vi "CommaScriptPaint.vi"(7 "Zoom Factor":sgl, 9 "Starting Pos":i16(slide)=128 scale=340.0..50.0, 10 "string 2":string, 11 "string":string) -> (2 "new picture":picture, 3 "Array":string[](array[string]))   [LabVIEW 2018]
panel:
  out "new picture out":picture
  out "Scaling Factor":dbl=1.07143 format="%#_13g"
  out "Height":u32
  out "Width":u32
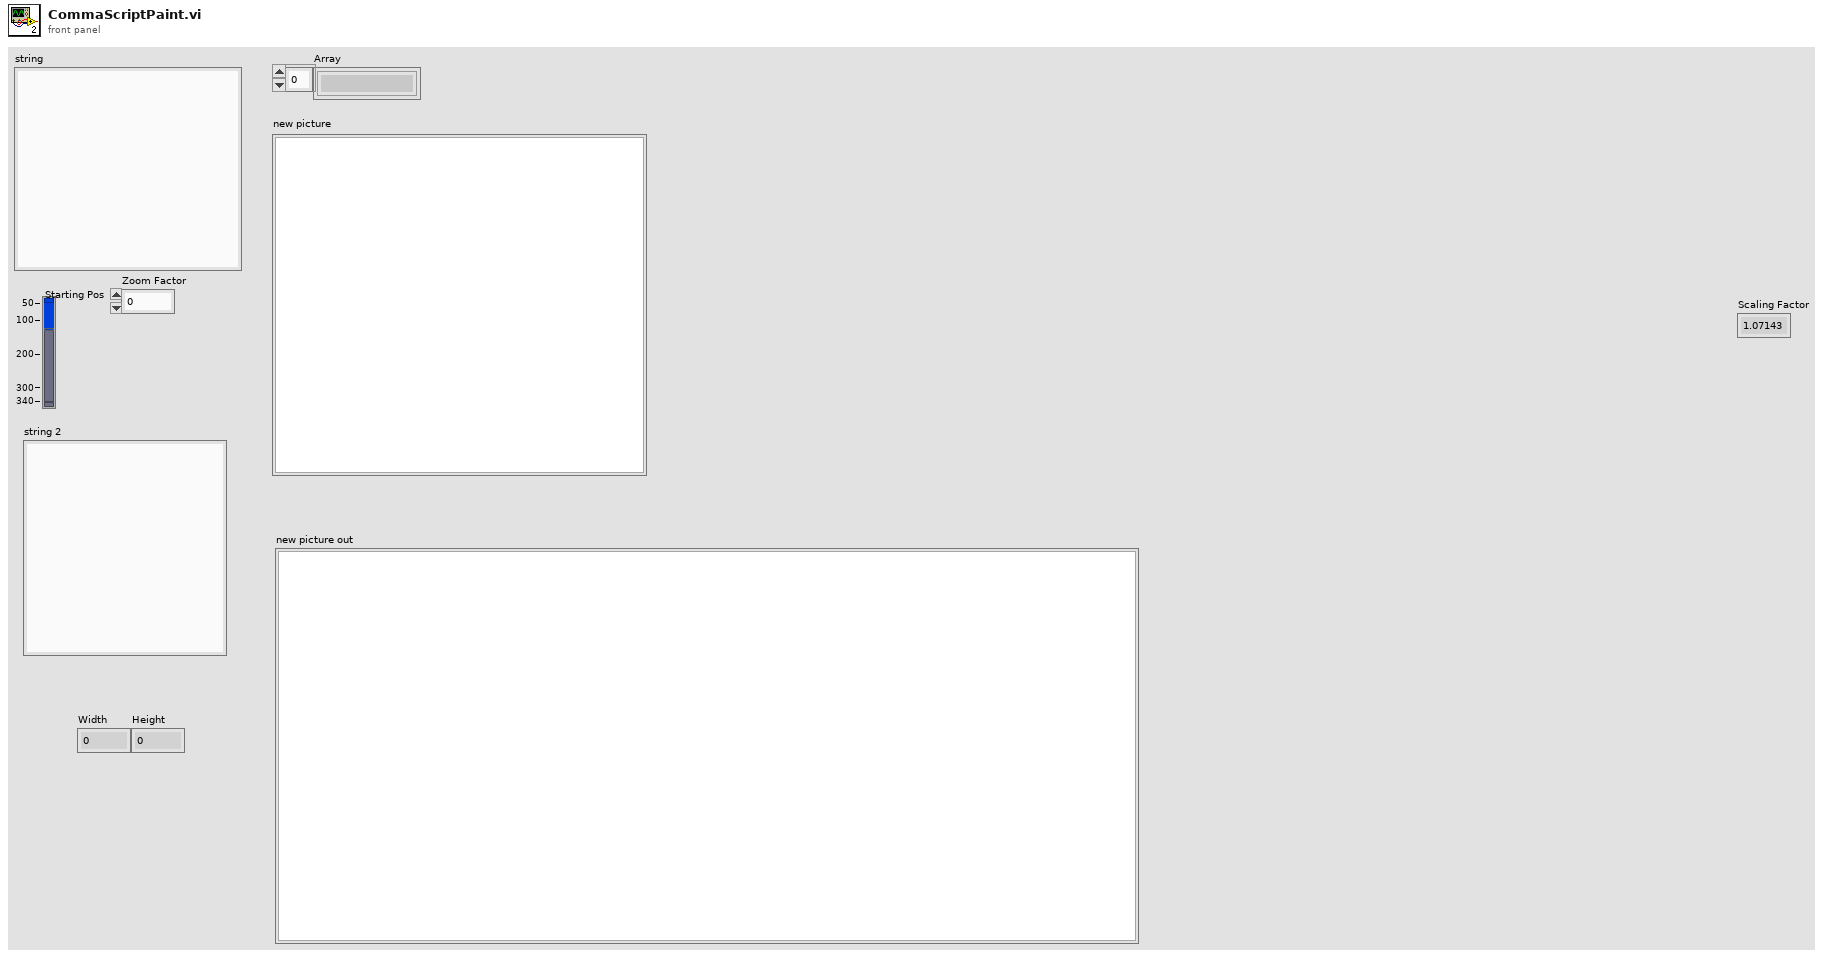
[diagram p1: front panel]
types:
  T1 = enum32{"invalid app kind", "Development System", "Run Time System", "Student Edition", "Embedded LabVIEW", "Evaluation", "Custom"}
  T2 = typedef "imagedata.ctl" = cluster{"image type":i32, "image depth":i32, "image":u8[], "mask":u8[], "colors":u32[], "Rectangle":cluster{"left":i16, "top":i16, "right":i16, "bottom":i16}}
  T3 = typedef "LVBoundsTypeDef.ctl" = cluster{"Width":u32, "Height":u32}
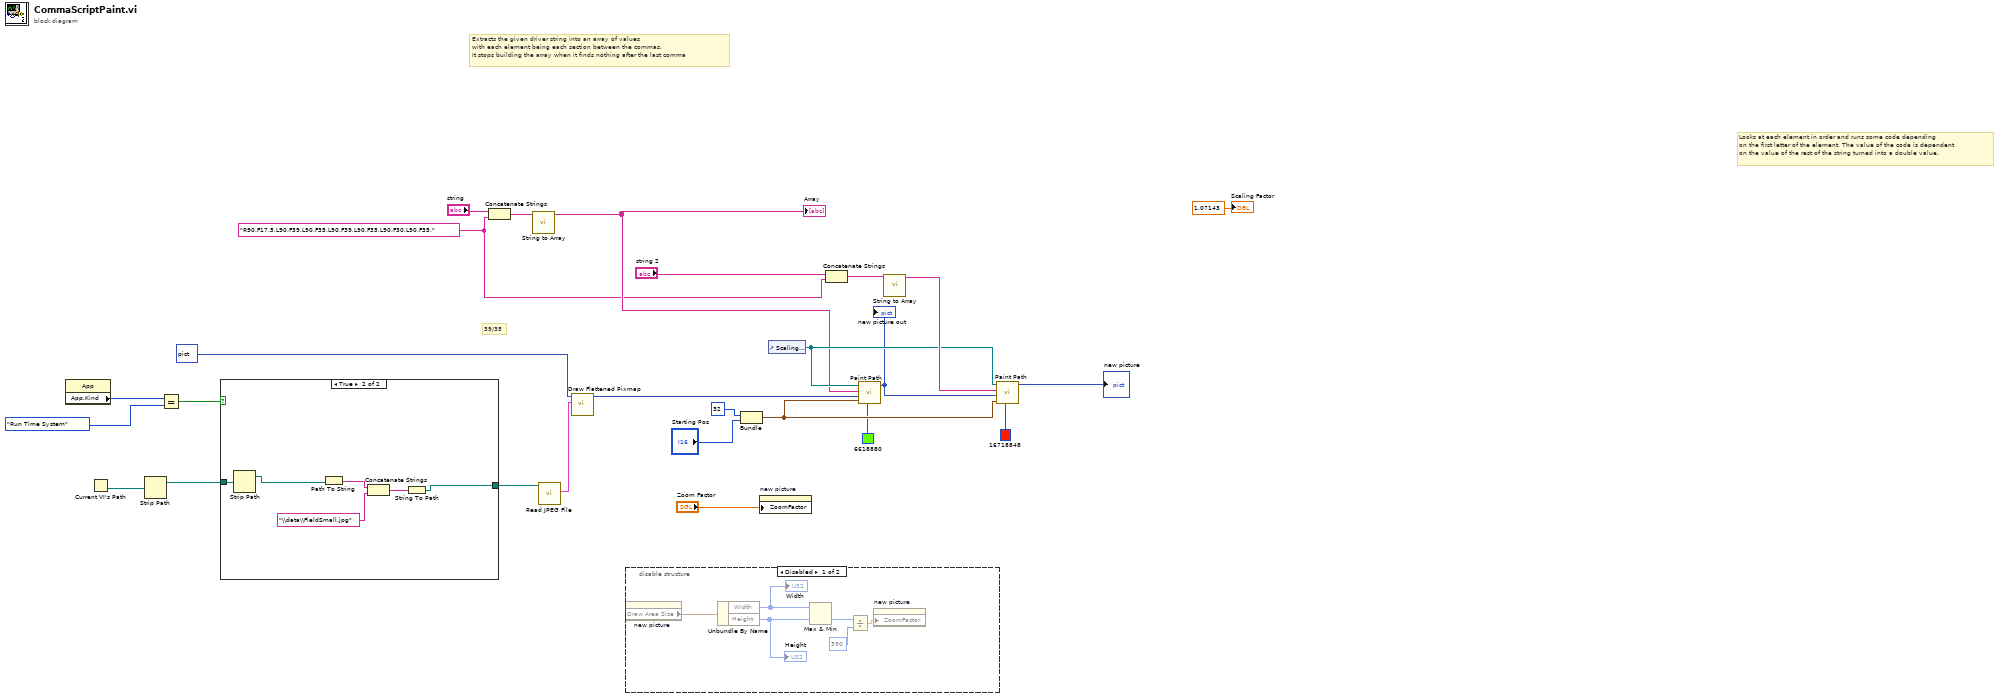
[diagram p0: block diagram]
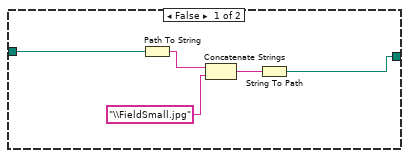
[diagram p3: hidden frame]
diagram:
  w1 = "R90,F17.5,L90,F39,L90,F35,L90,F39,L90,F35,L90,F30,L90,F35,"
  # "39/35"
  # "Extracts the given driver string into an array of values \nwith each element being each section between the commas.\nIt stops building the array when it finds nothing after the last comma"
  # "Looks at each element in order and runs some code depending\non the first letter of the element. The value of the code is dependent\non the value of the rest of the string turned into a double value."
  n1 = property class="App"() -> ("App.Kind"=w22:T1)  [unwired: 2 in, 2 out]
  n2 = Current VI's Path() -> (path=w19:path)
  n3 = Strip Path(path=w19) -> (stripped path=w20:path)  [unwired: 1 out]
  n4 = Equal?(x=w22, y=T1."Run Time System") -> (x = y?=w24:bool)
  n5 = case shown="True" w24 {
    tunnel: w20 -> [w29 w37]
    tunnel: [w27 w32] -> w25
    frame False {
      n6 = Path To String(path=w29) -> (string=w28:string)
      n7 = Concatenate Strings(w28, "\\FieldSmall.jpg" ("name or relative path")) -> (w31:string)
      n8 = String To Path(string=w31) -> (path=w27:path)
    }
    frame True {
      n9 = Strip Path(path=w37) -> (stripped path=w36:path)  [unwired: 1 out]
      n10 = Path To String(path=w36) -> (string=w35:string)
      n11 = Concatenate Strings(w35, "\\data\\FieldSmall.jpg" ("name or relative path")) -> (w33:string)
      n12 = String To Path(string=w33) -> (path=w32:path)
    }
  }
  n13 = Concatenate Strings("string", w1) -> (w4:string)
  n14 = call "String to Array.vi"("string"=w4) -> ("Array"=w6:string[])  [unwired: 10 in]
  "Array" <- w6
  n15 = call <vilib>:"Read JPEG File.vi"("path to JPEG file"=w25) -> ("image data"=w26:T2)  [unwired: 8 in, 2 out]
  n16 = call <vilib>:"Draw Flattened Pixmap.vi"("image data"=w26, "picture"=picture data[5B]) -> ("new picture"=w15:picture)  [unwired: 7 in]
  n17 = disable-structure shown="Disabled" {
    frame Disabled {
      n18 = property on="new picture" class="Pict"() -> ("Draw Area Size"=w39:T3)  [unwired: 2 in, 2 out]
      n19 = Unbundle By Name(w39) -> ("Width"=w43:u32, "Height"=w42:u32)
      "Width" <- w43
      "Height" <- w42
      n20 = Max & Min(x=w43, y=w42) -> (min(x,y)=w41:u32)  [unwired: 1 out]
      n21 = Divide(x=w41, y=u32 390) -> (x/y=w38:dbl)
      n22 = property on="new picture" class="Pict"("ZoomFactor"=w38) -> ()  [unwired: 2 in, 2 out]
    }
    frame Enabled {
    }
  }
  n23 = Bundle("x"=i16 32, "Starting Pos"="Starting Pos") -> (w11:cluster{"x":i16, "Starting Pos":i16})  [unwired: 1 in]
  n24 = property on="new picture" class="Pict"("ZoomFactor"="Zoom Factor") -> ()  [unwired: 2 in, 2 out]
  n25 = control-ref of="Scaling Factor"() -> (w13:refnum<vi>)
  n26 = Concatenate Strings("string 2", w1) -> (w2:string)
  n27 = call "Paint Path.vi"("color(Green)"=u32 6618880, "Starting Pos"=w11, "new picture in"=w15, "Array"=w6, "Digital in"=w13) -> ("new picture out"=w12:picture)  [unwired: 6 in]
  "new picture out" <- w12
  n28 = call "String to Array.vi"("string"=w2) -> ("Array"=w14:string[])  [unwired: 10 in]
  n29 = call "Paint Path.vi"("color(Green)"=u32 16718848, "Starting Pos"=w11, "new picture in"=w12, "Array"=w14, "Digital in"=w13) -> ("new picture out"=→"new picture":picture)  [unwired: 6 in]
  "Scaling Factor" <- 1.07143 ("Scaling Factor")
